vi "SubVI Tester.vi"() -> ()   [LabVIEW 2015]
panel:
  in  "Min Temperature":dbl=10.0
  in  "Max Temperature":dbl=30.0
  in  "Stop":bool
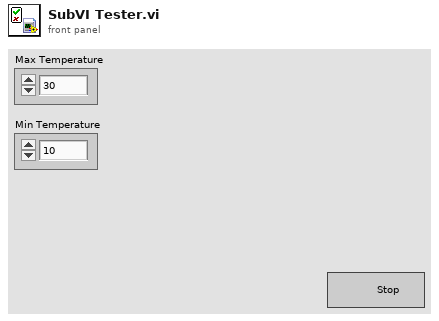
[diagram p1: front panel]
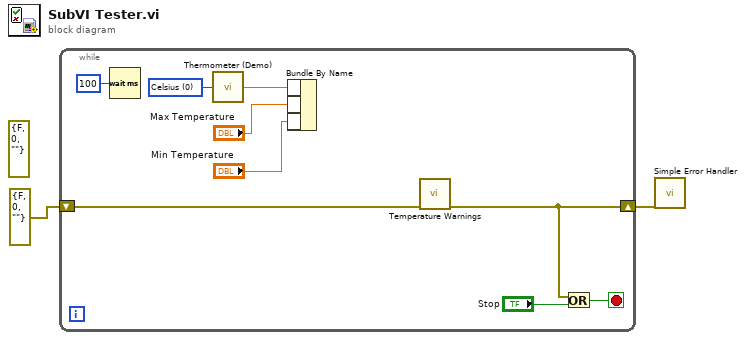
[diagram p0: block diagram]
diagram:
  (unwired) errorcluster {"status"=FALSE, "code"=0, "source"=""} ("error out")
  n1 = while {
    shift-right: [w7] -> w2
    shift-left: errorcluster {"status"=FALSE, "code"=0, "source"=""} ("error out") -> [w8]
    stop <- w9 stop-if-true
    w6 = u16 0 items=["Celsius", "Fahrenheit"] ("Units (0: Celsius)")
    n2 = Wait (ms)(milliseconds to wait=u32 100) -> ()  [unwired: 1 out]
    n3 = call "Thermometer (Demo).vi"("Units (0: Celsius)"=w6) -> ("Temperature Value"=w5:dbl)
    n4 = Bundle By Name(w5, "Max Temperature", "Min Temperature") -> ()  [unwired: 1 in, 1 out]
    n5 = call "Temperature Warnings.vi"("Error In"=w8) -> ("Error Out"=w7:errorcluster)  [unwired: 10 in]
    n6 = Or(x=w7, y="Stop") -> (x .or. y?=w9:bool)
  }
  n7 = call <vilib>:"Simple Error Handler.vi"("error in (no error)"=w2) -> ()  [unwired: 4 in, 5 out]
